vi "Start Task.vi"(8 "error in":errorcluster, 11 "Analog Input in":refnum<class "NI Analog Input.lvclass">) -> (0 "error out":errorcluster, 3 "Analog Input out":refnum<class "NI Analog Input.lvclass">)   [LabVIEW 2023, in "HardwareAbstractionLayer_LVOOP.lvlib" / "NI Analog Input.lvclass"]
doc: "This VI is DAQmx Start Task"
uses:
  NI Analog Input.lvclass
  NI Analog Input.lvclass/NI Analog Input.ctl
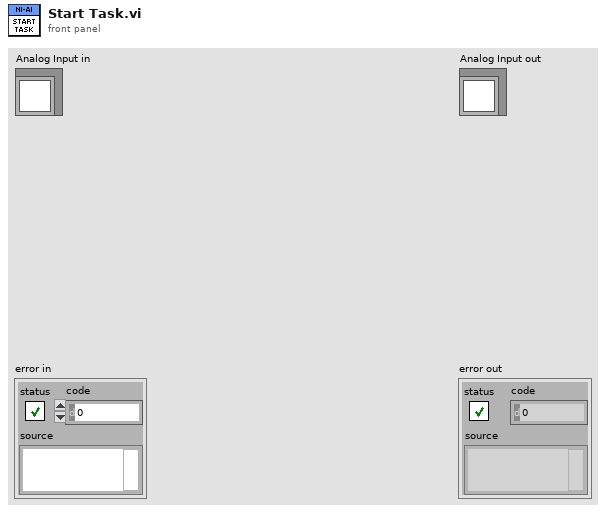
[diagram p1: front panel]
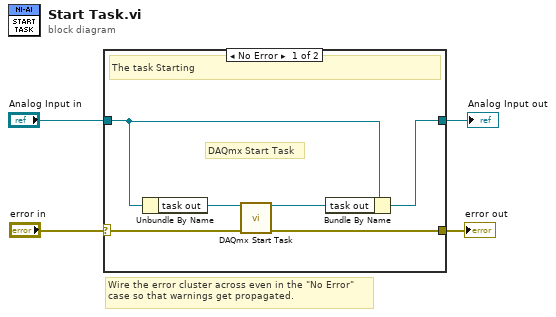
[diagram p0: block diagram]
diagram:
  # "Wire the error cluster across even in the \"No Error\"\ncase so that warnings get propagated."
  n1 = case shown="No Error" "error in" {
    selector: "error in" -> [w10 w12]
    tunnel: [w9 w12] -> w3
    tunnel: [w6 w11] -> w1
    tunnel: "Analog Input in" -> [w7 w11]
    frame No Error {
      # "DAQmx Start Task"
      # "The task Starting"
      n2 = Unbundle By Name(w7) -> ("task out"=w8:refnum<k21>)
      n3 = call <vilib>:"DAQmx Start Task.vi"("task/channels in"=w8, "error in"=w10) -> ("task out"=w5:refnum<k21>, "error out"=w9:errorcluster)  [unwired: 12 in]
      n4 = Bundle By Name(cluster=w7, "task out"=w5) -> (w6:refnum<class "NI Analog Input.lvclass">)
    }
    frame Error {
    }
  }
  "error out" <- w3
  "Analog Input out" <- w1
